vi "内置参数设置.vi"() -> ()   [LabVIEW 2016, in "斯坦道CODMn新电路板.lvlib"]
uses:
  <vilib>/Utility/miscctls.llb/LVPointTypeDef.ctl
panel:
  in  "是否存在液位检测板:":u16(ring) items=["否", "是"]
  in  "检出限(mg/L):":dbl
  in  "测量精度(mg/L):":dbl
  in  "ILimitDown":dbl
  in  "ILimitUp:":dbl
  in  "K d:":dbl
  in  "K i:":dbl
  in  "K p:":dbl
  in  "加热超时时间:(单位:秒)":dbl
  in  "告警温度:":dbl
  in  "加热温度:  校准参数":dbl
  in  "运行速度:  (修改需要重启)":u16
  in  "偏心轮: 校准参数":dbl
  in  "注射泵加热超时时间(s):":u16
  in  "注射泵保温温度H:":u8
  in  "注射泵保温温度L:":u8
  in  "废液通道:":u8
  in  "纯水通道:":u8
  in  "滴定速度:":u16
  in  "出样速度:":u16
  in  "进样速度:":u16
  in  "阀数量:":u8(ring) items=["9通"=9, "12通"=12]
  in  "注射泵型号":u8(ring) items=["TECAN", "润泽"]
  in  "阈值(高→低)(mg/L):":dbl
  in  "阈值(低→高)(mg/L):":dbl
  in  "检测下限(mg/L):":dbl
  in  "检测上限(mg/L):":dbl
  in  "关闭":bool
  in  "保存":bool
  in  "读取":bool
  # "仪器内部参数设置"
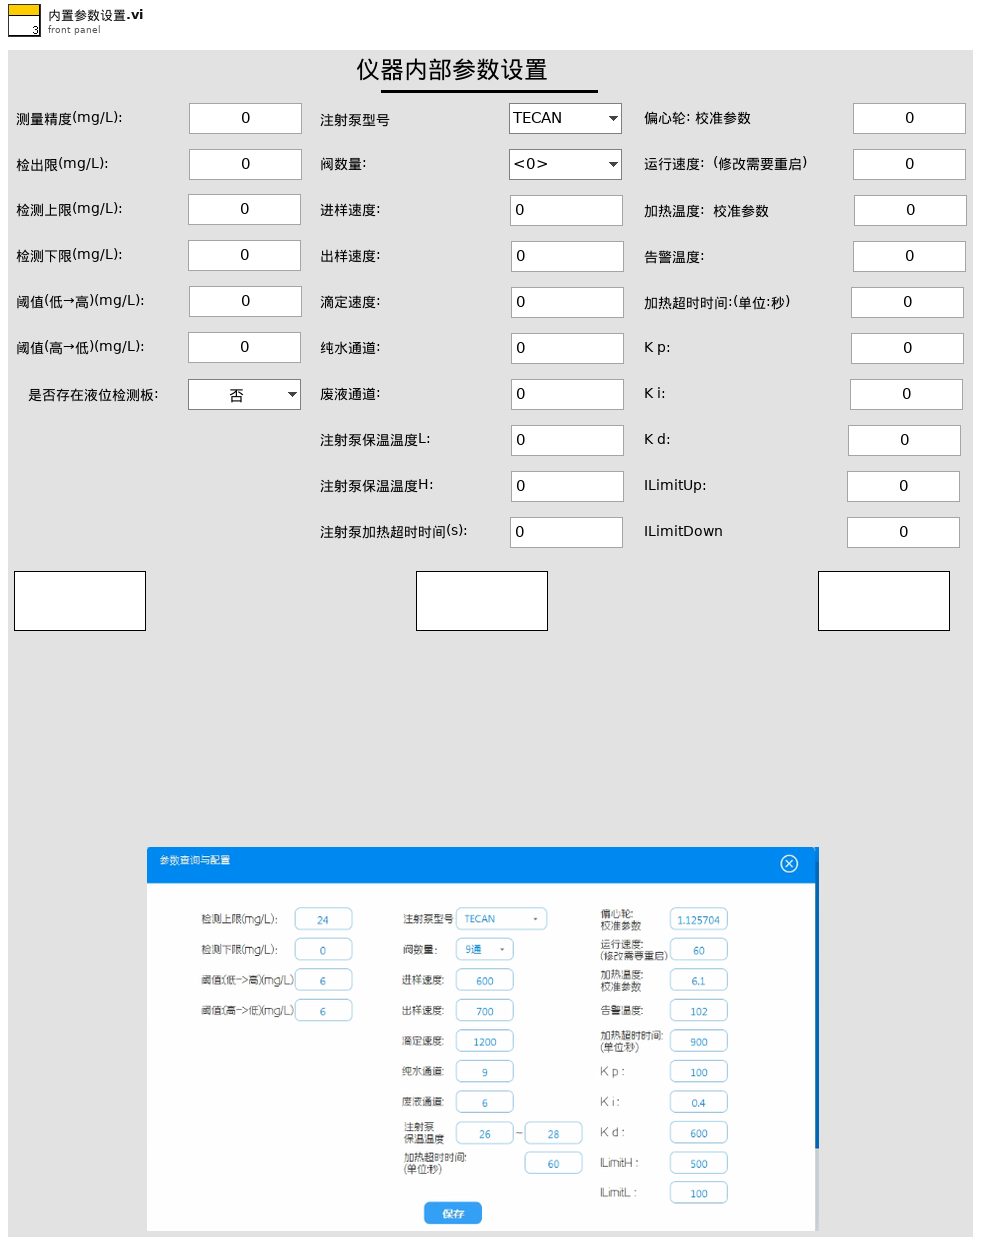
[diagram p1: front panel]
types:
  T1 = typedef "LVPointTypeDef.ctl" = cluster{"Horizontal":i16, "Vertical":i16}
  T2 = cluster{"偏心轮校准参数":dbl, "运行速度(修改需要重启)":u16, "加热温度(校准参数) ":dbl, "告警温度":dbl, "加热超时时间:(单位/秒)":dbl, "K p":dbl, "K i":dbl, "K d":dbl, "ILimitUp":dbl, "ILimitDown":dbl}
  T3 = cluster{"泵类型":u8, "阀数量":u8, "纯水通道":u8, "废液通道":u8, "进样速度":u16, "出样速度":u16, "滴定速度":u16, "注射泵保温温度L":u8, "注射泵保温温度H":u8, "注射泵加热超时时间":u16, "是否存在液位检测板":u16}
  T4 = cluster{"检出限":dbl, "测量精度":dbl, "上限":dbl, "下限":dbl, "阈值（低->高）":dbl, "阈值（高->低）":dbl}
  T5 = cluster{"测量精度":dbl, "检出限":dbl, "上限":dbl, "下限":dbl, "阈值（低->高）":dbl, "阈值（高->低）":dbl}
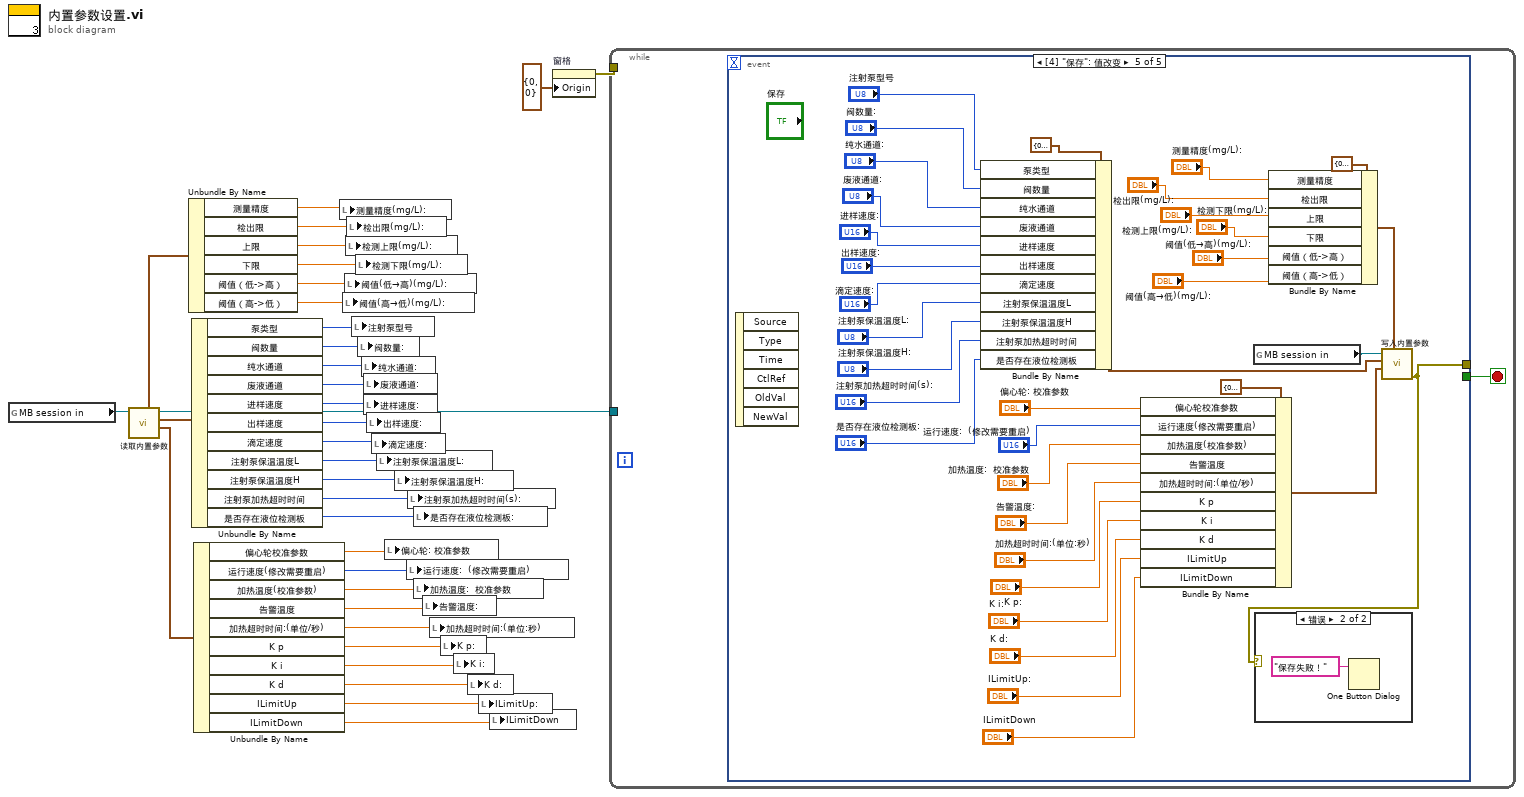
[diagram p0: block diagram]
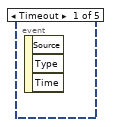
[diagram p2: hidden frame]
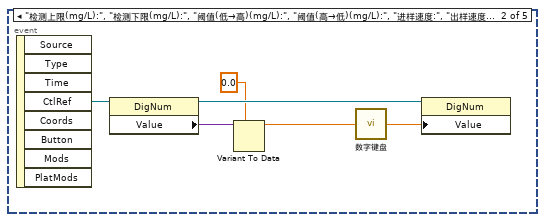
[diagram p3: hidden frame]
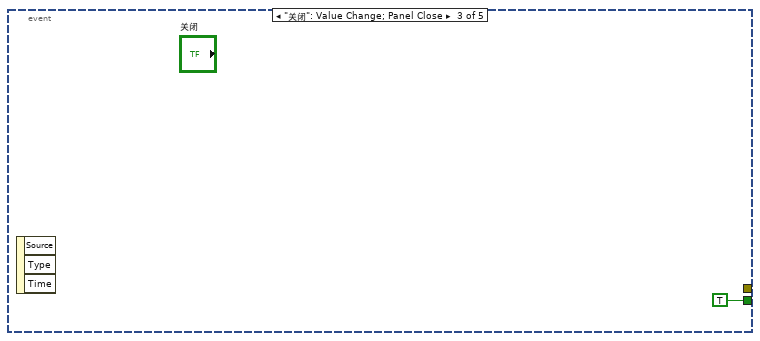
[diagram p4: hidden frame]
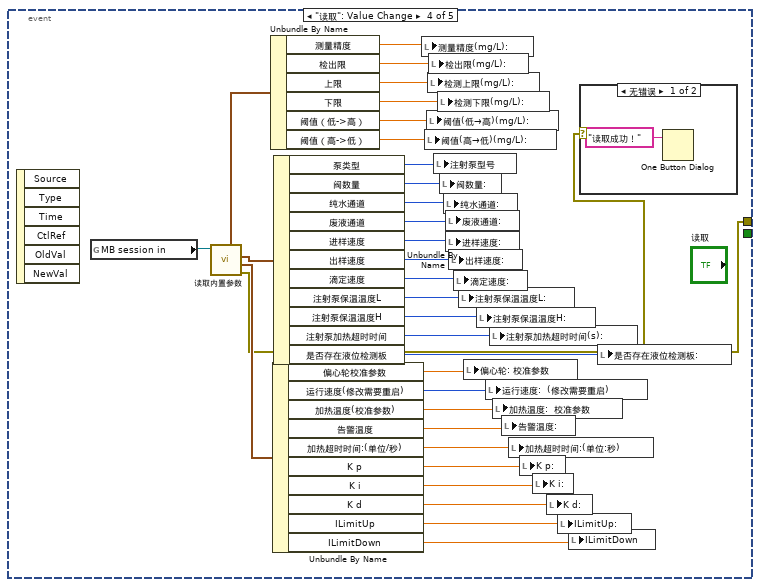
[diagram p5: hidden frame]
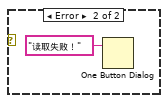
[diagram p6: hidden frame]
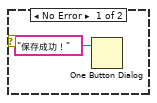
[diagram p7: hidden frame]
diagram:
  n1 = global read "VARCODMn全局变量.vi" "MB session in"() -> (w32:refnum<class "MB_Master.lvclass">)
  n2 = call "读取内置参数.vi"("MB session in"=w32) -> ("float"=w28:T2, "外设配置"=w29:T3, "MB session out"=w31:refnum<class "MB_Master.lvclass">, "量程参数读取"=w30:T4)  [unwired: 6 in, 1 out]
  n3 = Unbundle By Name(w30) -> ("测量精度"=w27:dbl, "检出限"=w26:dbl, "上限"=w25:dbl, "下限"=w24:dbl, "阈值（低->高）"=w23:dbl, "阈值（高->低）"=w22:dbl)
  n4 = Unbundle By Name(w29) -> ("泵类型"=w21:u8, "阀数量"=w20:u8, "纯水通道"=w19:u8, "废液通道"=w18:u8, "进样速度"=w17:u16, "出样速度"=w16:u16, "滴定速度"=w15:u16, "注射泵保温温度L"=w14:u8, "注射泵保温温度H"=w13:u8, "注射泵加热超时时间"=w12:u16, "是否存在液位检测板"=w1:u16)
  n5 = Unbundle By Name(w28) -> ("偏心轮校准参数"=w11:dbl, "运行速度(修改需要重启)"=w10:u16, "加热温度(校准参数)"=w9:dbl, "告警温度"=w8:dbl, "加热超时时间:(单位/秒)"=w7:dbl, "K p"=w6:dbl, "K i"=w5:dbl, "K d"=w4:dbl, "ILimitUp"=w3:dbl, "ILimitDown"=w2:dbl)
  n6 = local write "测量精度(mg/L):"(w27) -> ()
  n7 = local write "阈值(高→低)(mg/L):"(w22) -> ()
  n8 = local write "阈值(低→高)(mg/L):"(w23) -> ()
  n9 = local write "检测上限(mg/L):"(w25) -> ()
  n10 = local write "检出限(mg/L):"(w26) -> ()
  n11 = local write "注射泵型号"(w21) -> ()
  n12 = local write "检测下限(mg/L):"(w24) -> ()
  n13 = local write "阀数量:"(w20) -> ()
  n14 = local write "纯水通道:"(w19) -> ()
  n15 = local write "废液通道:"(w18) -> ()
  n16 = local write "进样速度:"(w17) -> ()
  n17 = local write "出样速度:"(w16) -> ()
  n18 = local write "滴定速度:"(w15) -> ()
  n19 = local write "注射泵保温温度L:"(w14) -> ()
  n20 = local write "偏心轮: 校准参数"(w11) -> ()
  n21 = local write "注射泵保温温度H:"(w13) -> ()
  n22 = local write "运行速度:  (修改需要重启)"(w10) -> ()
  n23 = local write "注射泵加热超时时间(s):"(w12) -> ()
  n24 = local write "是否存在液位检测板:"(w1) -> ()
  n25 = local write "加热温度:  校准参数"(w9) -> ()
  n26 = local write "告警温度:"(w8) -> ()
  n27 = local write "加热超时时间:(单位:秒)"(w7) -> ()
  n28 = local write "K p:"(w6) -> ()
  n29 = local write "K i:"(w5) -> ()
  n30 = local write "K d:"(w4) -> ()
  n31 = local write "ILimitUp:"(w3) -> ()
  n32 = local write "ILimitDown"(w2) -> ()
  n33 = property on="窗格" class="Pane"("Origin"=T1 {"Horizontal"=0, "Vertical"=0} ("原点")) -> (error out=w33:errorcluster)  [unwired: 2 in, 1 out]
  n34 = while {
    tunnel: w33 -> [_]
    tunnel: w31 -> [_]
    stop <- w35 stop-if-true
    n35 = event shown="[4] \"保存\": 值改变" {
      selector: _ -> [_ _ _ _ _]
      dyn-events: _ -> [_ _ _ _ _]
      timeout: _ -> [_ _ _ _ _]
      tunnel: [_ _ TRUE _ _] -> w35
      tunnel: [_ _ _ w44 w79] -> _
      event Timeout {
        n36 = event-data() -> ()  [unwired: 1 in, 3 out]
      }
      event "检测上限(mg/L):", "检测下限(mg/L):", "阈值(低→高)(mg/L):", "阈值(高→低)(mg/L):", "进样速度:", "出样速度:", "滴定速度:", "纯水通道:", "废液通道:", "注射泵保温温度L:", "注射泵保温温度H:", "注射泵加热超时时间(s):", "偏心轮: 校准参数", "运行速度:  (修改需要重启)", "告警温度:", "加热温度:  校准参数", "K p:", "K i:", "K d:", "ILimitUp:", "ILimitDown", "测量精度(mg/L):", "检出限(mg/L):": Mouse Down {
        n37 = event-data() -> ("CtlRef"=w41:refnum<vi>)  [unwired: 1 in, 7 out]
        n38 = property class="DigNum"(reference=w41) -> (reference out=w40:refnum<vi>, "Value"=w38:variant)  [unwired: 1 in, 1 out]
        n39 = Variant To Data(type=0.0 ("OldNumber"), Variant=w38) -> (data=w36:dbl)  [unwired: 1 in, 1 out]
        n40 = call "数字键盘.vi"("OldNumber"=w36) -> ("NewNumber"=w39:dbl)
        n41 = property class="DigNum"(reference=w40, "Value"=w39) -> ()  [unwired: 1 in, 2 out]
      }
      event "关闭": Value Change; Panel Close {
        n42 = event-data() -> ()  [unwired: 1 in, 3 out]
      }
      event "读取": Value Change {
        n43 = event-data() -> ()  [unwired: 1 in, 6 out]
        n44 = global read "VARCODMn全局变量.vi" "MB session in"() -> (w45:refnum<class "MB_Master.lvclass">)
        n45 = call "读取内置参数.vi"("MB session in"=w45) -> ("error out"=w44:errorcluster, "float"=w48:T2, "外设配置"=w47:T3, "量程参数读取"=w46:T4)  [unwired: 6 in, 1 out]
        n46 = Unbundle By Name(w46) -> ("测量精度"=w49:dbl, "检出限"=w50:dbl, "上限"=w51:dbl, "下限"=w52:dbl, "阈值（低->高）"=w53:dbl, "阈值（高->低）"=w54:dbl)
        n47 = Unbundle By Name(w48) -> ("偏心轮校准参数"=w65:dbl, "运行速度(修改需要重启)"=w66:u16, "加热温度(校准参数)"=w67:dbl, "告警温度"=w68:dbl, "加热超时时间:(单位/秒)"=w69:dbl, "K p"=w70:dbl, "K i"=w71:dbl, "K d"=w72:dbl, "ILimitUp"=w73:dbl, "ILimitDown"=w74:dbl)
        n48 = Unbundle By Name(w47) -> ("泵类型"=w55:u8, "阀数量"=w56:u8, "纯水通道"=w57:u8, "废液通道"=w58:u8, "进样速度"=w59:u16, "出样速度"=w60:u16, "滴定速度"=w61:u16, "注射泵保温温度L"=w62:u8, "注射泵保温温度H"=w63:u8, "注射泵加热超时时间"=w64:u16, "是否存在液位检测板"=w43:u16)
        n49 = local write "测量精度(mg/L):"(w49) -> ()
        n50 = local write "阈值(高→低)(mg/L):"(w54) -> ()
        n51 = local write "阈值(低→高)(mg/L):"(w53) -> ()
        n52 = local write "检测上限(mg/L):"(w51) -> ()
        n53 = local write "检出限(mg/L):"(w50) -> ()
        n54 = local write "注射泵型号"(w55) -> ()
        n55 = local write "检测下限(mg/L):"(w52) -> ()
        n56 = local write "阀数量:"(w56) -> ()
        n57 = local write "纯水通道:"(w57) -> ()
        n58 = local write "废液通道:"(w58) -> ()
        n59 = local write "进样速度:"(w59) -> ()
        n60 = local write "出样速度:"(w60) -> ()
        n61 = local write "滴定速度:"(w61) -> ()
        n62 = local write "注射泵保温温度L:"(w62) -> ()
        n63 = local write "偏心轮: 校准参数"(w65) -> ()
        n64 = local write "注射泵保温温度H:"(w63) -> ()
        n65 = local write "运行速度:  (修改需要重启)"(w66) -> ()
        n66 = local write "注射泵加热超时时间(s):"(w64) -> ()
        n67 = local write "加热温度:  校准参数"(w67) -> ()
        n68 = local write "告警温度:"(w68) -> ()
        n69 = local write "加热超时时间:(单位:秒)"(w69) -> ()
        n70 = local write "K p:"(w70) -> ()
        n71 = local write "K i:"(w71) -> ()
        n72 = local write "K d:"(w72) -> ()
        n73 = local write "ILimitUp:"(w73) -> ()
        n74 = local write "ILimitDown"(w74) -> ()
        n75 = case shown="无错误" w44 {
          frame No Error {
            n76 = One Button Dialog(message="读取成功！" ("消息")) -> ()  [unwired: 1 in, 1 out]
          }
          frame Error {
            n77 = One Button Dialog(message="读取失败！" ("消息")) -> ()  [unwired: 1 in, 1 out]
          }
        }
        n78 = local write "是否存在液位检测板:"(w43) -> ()
      }
      event "保存": Value Change {
        n79 = event-data() -> ()  [unwired: 1 in, 6 out]
        n80 = Bundle By Name(cluster=T3 {"泵类型"=0, "阀数量"=0, "纯水通道"=0, "废液通道"=0, "进样速度"=0, "出样速度"=0, "滴定速度"=0, "注射泵保温温度L"=0, "注射泵保温温度H"=0, "注射泵加热超时时间"=0, "是否存在液位检测板"=0} ("外设配置"), "泵类型"="注射泵型号", "阀数量"="阀数量:", "纯水通道"="纯水通道:", "废液通道"="废液通道:", "进样速度"="进样速度:", "出样速度"="出样速度:", "滴定速度"="滴定速度:", "注射泵保温温度L"="注射泵保温温度L:", "注射泵保温温度H"="注射泵保温温度H:", "注射泵加热超时时间"="注射泵加热超时时间(s):", "是否存在液位检测板"="是否存在液位检测板:") -> (w92:T3)
        n81 = Bundle By Name(cluster=T2 {"偏心轮校准参数"=0.0, "运行速度(修改需要重启)"=0, "加热温度(校准参数) "=0.0, "告警温度"=0.0, "加热超时时间:(单位/秒)"=0.0, "K p"=0.0, "K i"=0.0, "K d"=0.0, "ILimitUp"=0.0, "ILimitDown"=0.0} ("float"), "偏心轮校准参数"="偏心轮: 校准参数", "运行速度(修改需要重启)"="运行速度:  (修改需要重启)", "加热温度(校准参数)"="加热温度:  校准参数", "告警温度"="告警温度:", "加热超时时间:(单位/秒)"="加热超时时间:(单位:秒)", "K p"="K p:", "K i"="K i:", "K d"="K d:", "ILimitUp"="ILimitUp:", "ILimitDown"="ILimitDown") -> (w80:T2)
        n82 = global read "VARCODMn全局变量.vi" "MB session in"() -> (w111:refnum<class "MB_Master.lvclass">)
        n83 = Bundle By Name(cluster=T5 {"测量精度"=0.0, "检出限"=0.0, "上限"=0.0, "下限"=0.0, "阈值（低->高）"=0.0, "阈值（高->低）"=0.0} ("量程参数读取"), "测量精度"="测量精度(mg/L):", "检出限"="检出限(mg/L):", "上限"="检测上限(mg/L):", "下限"="检测下限(mg/L):", "阈值（低->高）"="阈值(低→高)(mg/L):", "阈值（高->低）"="阈值(高→低)(mg/L):") -> (w103:T5)
        n84 = call "写入内置参数.vi"("量程参数读取"=w103, "float"=w80, "外设配置"=w92, "MB session in"=w111) -> ("error out"=w79:errorcluster)  [unwired: 6 in, 1 out]
        n85 = case shown="错误" w79 {
          frame No Error {
            n86 = One Button Dialog(message="保存成功！" ("消息")) -> ()  [unwired: 1 in, 1 out]
          }
          frame Error {
            n87 = One Button Dialog(message="保存失败！" ("消息")) -> ()  [unwired: 1 in, 1 out]
          }
        }
      }
    }
  }
